vi "定时设置读取.vi"(11 "引用参数":string) -> (3 "周期设置输出":T6={"周期模式"=enum."不启用", "定点周期"={"启动命令"=0, "启动命令 2"=0, "启动命令 3"=0, "启动命令 4"=0, "启动命令 5"=0, "启动命令 6"=0, "启动命令 7"=0, "启动命令 8"=0, "启动命令 9"=0, "启动命令 10"=0, "启动命令 11"=0, "启动命令 12"=0, "启动命令 13"=0, "启动命令 14"=0, "启动命令 15"=0, "启动命令 16"=0, "启动命令 17"=0, "启动命令 18"=0, "启动命令 19"=0, "启动命令 20"=0, "启动命令 21"=0, "启动命令 22"=0, "启动命令 23"=0, "启动命令 24"=0}, "间隔启动"={"启动命令"=0, "启动间隔"=0.0, "启动次数"=0}, "测量参数"={"氨氮"=TRUE, "总磷"=TRUE, "总氮"=TRUE, "CODMn"=TRUE, "CODCr"=TRUE}} {"定点周期"."启动命令 24" items=["", "加标回收（启动采配水）", "加标回收（不启动采配水）", "水样测试（启动采配水）", "水样测试（不启动采配水）"]; "定点周期"."启动命令 23" items=["", "加标回收（启动采配水）", "加标回收（不启动采配水）", "水样测试（启动采配水）", "水样测试（不启动采配水）"]; "定点周期"."启动命令 22" items=["", "加标回收（启动采配水）", "加标回收（不启动采配水）", "水样测试（启动采配水）", "水样测试（不启动采配水）"]; "定点周期"."启动命令 21" items=["", "加标回收（启动采配水）", "加标回收（不启动采配水）", "水样测试（启动采配水）", "水样测试（不启动采配水）"]; "定点周期"."启动命令 20" items=["", "加标回收（启动采配水）", "加标回收（不启动采配水）", "水样测试（启动采配水）", "水样测试（不启动采配水）"]; "定点周期"."启动命令 19" items=["", "加标回收（启动采配水）", "加标回收（不启动采配水）", "水样测试（启动采配水）", "水样测试（不启动采配水）"]; "定点周期"."启动命令 18" items=["", "加标回收（启动采配水）", "加标回收（不启动采配水）", "水样测试（启动采配水）", "水样测试（不启动采配水）"]; "定点周期"."启动命令 17" items=["", "加标回收（启动采配水）", "加标回收（不启动采配水）", "水样测试（启动采配水）", "水样测试（不启动采配水）"]; "定点周期"."启动命令 16" items=["", "加标回收（启动采配水）", "加标回收（不启动采配水）", "水样测试（启动采配水）", "水样测试（不启动采配水）"]; "定点周期"."启动命令 15" items=["", "加标回收（启动采配水）", "加标回收（不启动采配水）", "水样测试（启动采配水）", "水样测试（不启动采配水）"]; "定点周期"."启动命令 14" items=["", "加标回收（启动采配水）", "加标回收（不启动采配水）", "水样测试（启动采配水）", "水样测试（不启动采配水）"]; "定点周期"."启动命令 13" items=["", "加标回收（启动采配水）", "加标回收（不启动采配水）", "水样测试（启动采配水）", "水样测试（不启动采配水）"]; "定点周期"."启动命令 12" items=["", "加标回收（启动采配水）", "加标回收（不启动采配水）", "水样测试（启动采配水）", "水样测试（不启动采配水）"]; "定点周期"."启动命令 11" items=["", "加标回收（启动采配水）", "加标回收（不启动采配水）", "水样测试（启动采配水）", "水样测试（不启动采配水）"]; "定点周期"."启动命令 10" items=["", "加标回收（启动采配水）", "加标回收（不启动采配水）", "水样测试（启动采配水）", "水样测试（不启动采配水）"]; "定点周期"."启动命令 9" items=["", "加标回收（启动采配水）", "加标回收（不启动采配水）", "水样测试（启动采配水）", "水样测试（不启动采配水）"]; "定点周期"."启动命令 8" items=["", "加标回收（启动采配水）", "加标回收（不启动采配水）", "水样测试（启动采配水）", "水样测试（不启动采配水）"]; "定点周期"."启动命令 7" items=["", "加标回收（启动采配水）", "加标回收（不启动采配水）", "水样测试（启动采配水）", "水样测试（不启动采配水）"]; "定点周期"."启动命令 6" items=["", "加标回收（启动采配水）", "加标回收（不启动采配水）", "水样测试（启动采配水）", "水样测试（不启动采配水）"]; "定点周期"."启动命令 5" items=["", "加标回收（启动采配水）", "加标回收（不启动采配水）", "水样测试（启动采配水）", "水样测试（不启动采配水）"]; "定点周期"."启动命令 4" items=["", "加标回收（启动采配水）", "加标回收（不启动采配水）", "水样测试（启动采配水）", "水样测试（不启动采配水）"]; "定点周期"."启动命令 3" items=["", "加标回收（启动采配水）", "加标回收（不启动采配水）", "水样测试（启动采配水）", "水样测试（不启动采配水）"]; "定点周期"."启动命令 2" items=["", "加标回收（启动采配水）", "加标回收（不启动采配水）", "水样测试（启动采配水）", "水样测试（不启动采配水）"]; "定点周期"."启动命令" items=["", "加标回收（启动采配水）", "加标回收（不启动采配水）", "水样测试（启动采配水）", "水样测试（不启动采配水）"]; "间隔启动"."启动命令" items=["", "加标回收（启动采配水）", "加标回收（不启动采配水）", "水样测试（启动采配水）", "水样测试（不启动采配水）"]})   [LabVIEW 2016, in "ZK定时设置.xctl"]
uses:
  <vilib>/Utility/config.llb/NI_LVConfig.lvlib
panel:
  # "分钟"
  # "次"
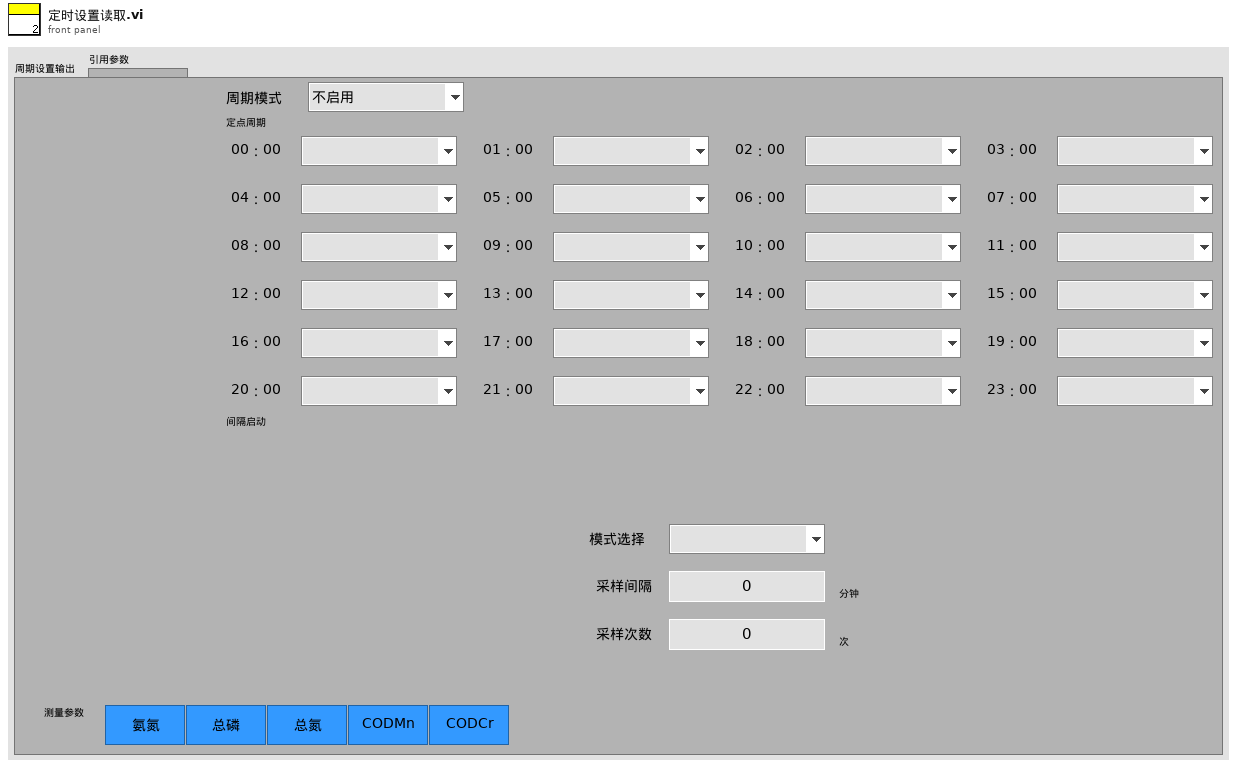
[diagram p1: front panel]
types:
  T1 = typedef "ZK定时设置.xctl/周期模式设置.ctl" = enum16{"不启用", "定点模式", "间隔模式"}
  T2 = typedef "ZK定时设置.xctl/定点周期设置.ctl" = cluster{"启动命令":T3, "启动命令 2":T3, "启动命令 3":T3, "启动命令 4":T3, "启动命令 5":T3, "启动命令 6":T3, "启动命令 7":T3, "启动命令 8":T3, "启动命令 9":T3, "启动命令 10":T3, "启动命令 11":T3, "启动命令 12":T3, "启动命令 13":T3, "启动命令 14":T3, "启动命令 15":T3, "启动命令 16":T3, "启动命令 17":T3, "启动命令 18":T3, "启动命令 19":T3, "启动命令 20":T3, "启动命令 21":T3, "启动命令 22":T3, "启动命令 23":T3, "启动命令 24":T3}
  T3 = typedef "ZK定时设置.xctl/启动命令选择.ctl" = u16
  T4 = typedef "ZK定时设置.xctl/间隔启动设置.ctl" = cluster{"启动命令":T3, "启动间隔":dbl, "启动次数":i32}
  T5 = typedef "ZK定时设置.xctl/测量参数.ctl" = cluster{"氨氮":bool, "总磷":bool, "总氮":bool, "CODMn":bool, "CODCr":bool}
  T6 = cluster{"周期模式":T1, "定点周期":T2, "间隔启动":T4, "测量参数":T5}
  T7 = typedef "NI_LVConfig.lvlib/Config Data RefNum.ctl" = refnum<k1>
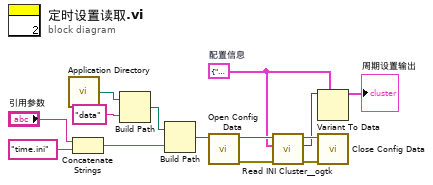
[diagram p0: block diagram]
diagram:
  w1 = T6 {"周期模式"=enum."不启用", "定点周期"={"启动命令"=0, "启动命令 2"=0, "启动命令 3"=0, "启动命令 4"=0, "启动命令 5"=0, "启动命令 6"=0, "启动命令 7"=0, "启动命令 8"=0, "启动命令 9"=0, "启动命令 10"=0, "启动命令 11"=0, "启动命令 12"=0, "启动命令 13"=0, "启动命令 14"=0, "启动命令 15"=0, "启动命令 16"=0, "启动命令 17"=0, "启动命令 18"=0, "启动命令 19"=0, "启动命令 20"=0, "启动命令 21"=0, "启动命令 22"=0, "启动命令 23"=0, "启动命令 24"=0}, "间隔启动"={"启动命令"=0, "启动间隔"=0.0, "启动次数"=0}, "测量参数"={"氨氮"=TRUE, "总磷"=TRUE, "总氮"=TRUE, "CODMn"=TRUE, "CODCr"=TRUE}}  # 配置信息
  n1 = call <vilib>:"Application Directory.vi"() -> ("Application Directory"=w14:path)
  n2 = Concatenate Strings("引用参数", "time.ini" ("名称或相对路径")) -> (w6:string)
  n3 = Build Path(base path=w14, name or relative path="data" ("名称或相对路径")) -> (appended path=w8:path)
  n4 = Build Path(base path=w8, name or relative path=w6) -> (appended path=w5:path)
  n5 = call <vilib>:"Open Config Data.vi"("configuration file path"=w5) -> ("error out"=w10:errorcluster, "refnum"=w12:T7)  [unwired: 8 in, 1 out]
  n6 = call <userlib>:"Read INI Cluster__ogtk.vi"("error in (no error)"=w10, "INI Fomatted Cluster Type"=w1, "refnum"=w12) -> ("error out"=w9:errorcluster, "INI Fomatted Cluster"=w4:variant, "dup refnum"=w11:T7)  [unwired: 4 in, 2 out]
  n7 = Variant To Data(type=w1, Variant=w4) -> (data=→"周期设置输出":T6)  [unwired: 1 in, 1 out]
  n8 = call <vilib>:"Close Config Data.vi"("error in (no error)"=w9, "refnum"=w11) -> ()  [unwired: 8 in, 2 out]
